vi "run.update_set_name.vi"(8 "error in":errorcluster, 11 "RunUpdateStaging in":refnum<class "RunUpdateStaging.lvclass">) -> (0 "error out":errorcluster, 3 "RunUpdateStaging out":refnum<class "RunUpdateStaging.lvclass">)   [LabVIEW 2020, in "RunUpdateStaging.lvclass"]
doc: "Stages a new name for the run being updated."
uses:
  RunUpdateStaging.lvclass
  RunUpdateStaging.lvclass/RunUpdateStaging.ctl
  client.lvlib
panel:
  in  "name":string
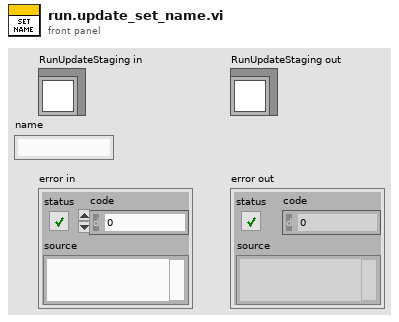
[diagram p1: front panel]
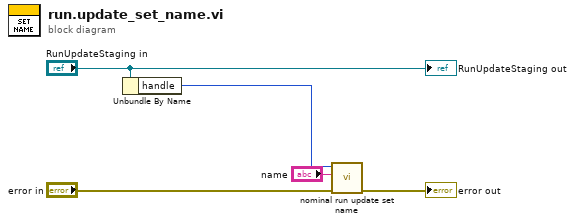
[diagram p0: block diagram]
diagram:
  n1 = Unbundle By Name("RunUpdateStaging in") -> ("handle"=w3:i32)
  n2 = call "nominal run update set name.vi"("error in (no error)"="error in", "name"="name", "staging"=w3) -> ("error out"=→"error out":errorcluster)  [unwired: 7 in, 1 out]
  "RunUpdateStaging out" <- "RunUpdateStaging in"
